vi "Parse URI.vi"(8 "error in (no error)":errorcluster, 11 "URI":string) -> (0 "error out":errorcluster, 3 "parsed URI":T1)   [LabVIEW 2020, in "NI_WFCN.lvlib"]
doc: "Parse a URI into its constituent parts. Component prefixes and suffixes denote presence:\n<b>suffixed user</b> ends with \"@\" if specified.\n<b>prefixed port</b> starts with \":\" if specified.\n<b>prefixed query</b> starts with \"?\" if specified.\n<b>prefixed fragment</b> starts with \"#\" if specified.\nIf a bare hostname is passed in, it will be returned in <b>undecoded.path</b>."
uses:
  <vilib>/net/WFCN/NI_WFCN.lvlib
  <vilib>/net/WFCN/Utility/URIv1.ctl
  <vilib>/net/WFCN/Utility/URI Path Components v1.ctl
  <vilib>/net/WFCN/Utility/URI Undecoded Components v1.ctl
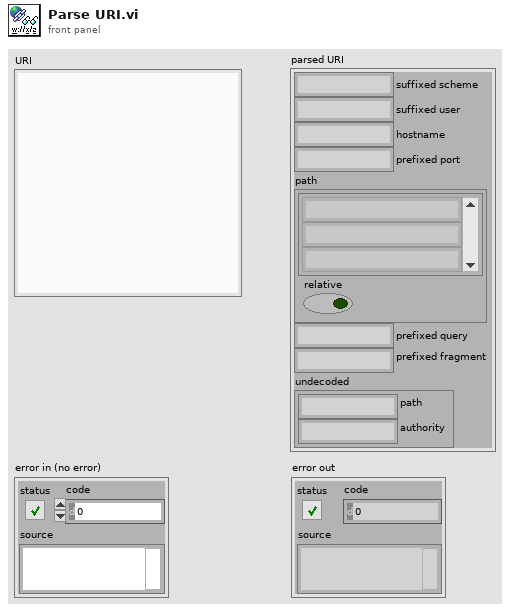
[diagram p1: front panel]
types:
  T1 = typedef "NI_WFCN.lvlib/URIv1.ctl" = cluster{"suffixed scheme":string, "suffixed user":string, "hostname":string, "prefixed port":string, "path":T2, "prefixed query":string, "prefixed fragment":string, "undecoded":T3}
  T2 = typedef "NI_WFCN.lvlib/URI Path Components v1.ctl" = cluster{"elements":string[], "relative":bool}
  T3 = typedef "NI_WFCN.lvlib/URI Undecoded Components v1.ctl" = cluster{"path":string, "authority":string}
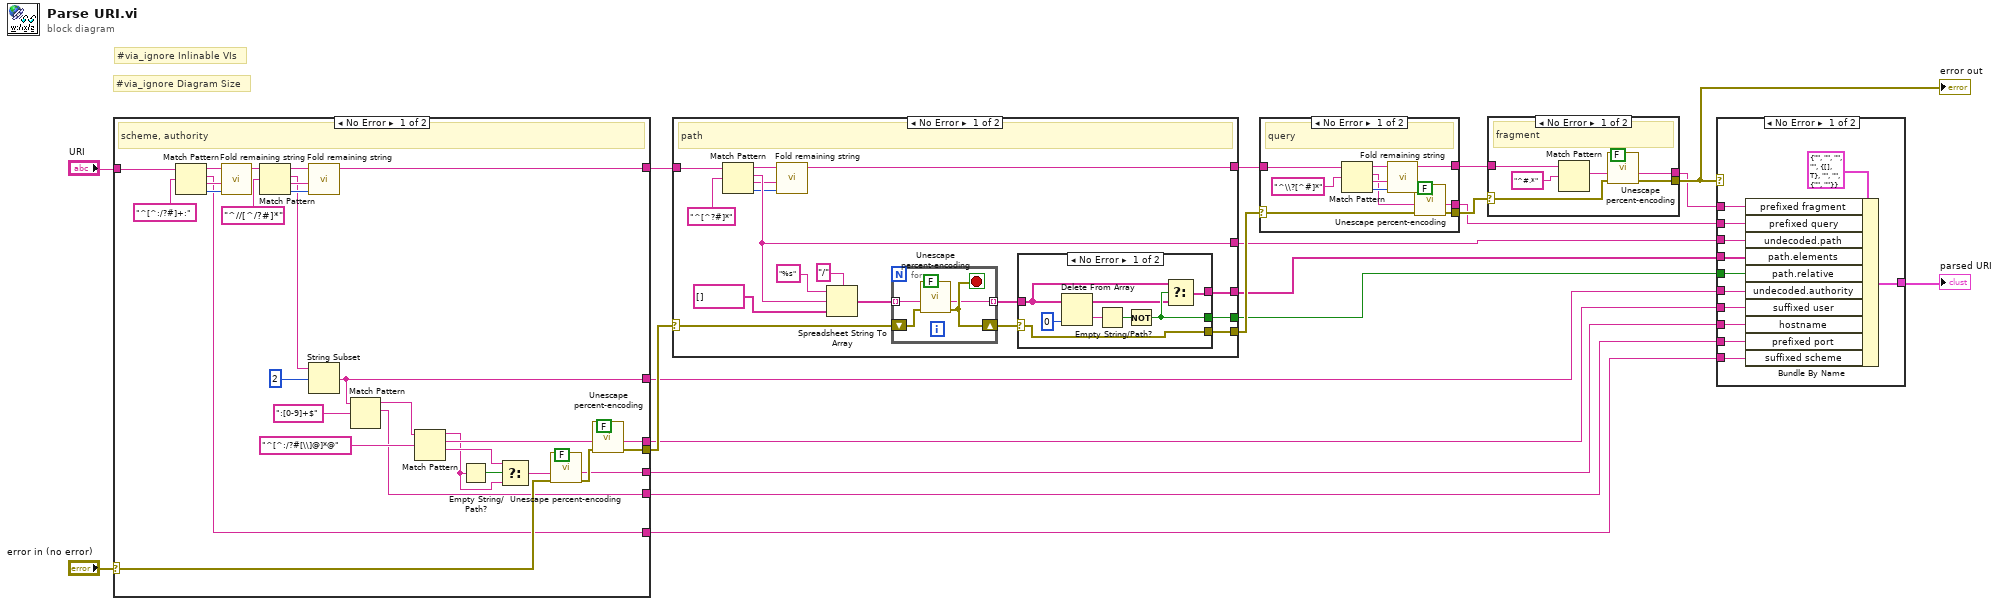
[diagram p0: block diagram]
diagram:
  # "#via_ignore Inlinable VIs"
  # "#via_ignore Diagram Size"
  n1 = case shown="No Error" "error in (no error)" {
    selector: "error in (no error)" -> [w32 w52]
    tunnel: "URI" -> [w51 _]
    tunnel: [w31 _] -> w15
    tunnel: [w30 w52] -> w16
    tunnel: [w29 _] -> w4
    tunnel: [w28 _] -> w3
    tunnel: [w27 _] -> w1
    tunnel: [w26 _] -> w2
    tunnel: [w25 _] -> w5
    frame No Error {
      # "scheme, authority"
      n2 = Match Pattern(string=w51, regular expression="^[^:/?#]+:") -> (before substring=w46:string, match substring=w27:string, after substring=w45:string, offset past match=w44:i32)  [unwired: 1 in]
      n3 = call <vilib>:"Fold remaining string.vi"("index"=w44, "after match"=w45, "before match"=w46) -> ("remaining"=w43:string)  [unwired: 4 in]
      n4 = Match Pattern(string=w43, regular expression="^//[^/?#]*") -> (before substring=w41:string, match substring=w37:string, after substring=w40:string, offset past match=w39:i32)  [unwired: 1 in]
      n5 = call <vilib>:"Fold remaining string.vi"("index"=w39, "after match"=w40, "before match"=w41) -> ("remaining"=w31:string)  [unwired: 4 in]
      n6 = String Subset(string=w37, offset (0)=2) -> (substring=w25:string)  [unwired: 1 in]
      n7 = Match Pattern(string=w25, regular expression=":[0-9]+$") -> (before substring=w48:string, match substring=w26:string)  [unwired: 1 in, 2 out]
      n8 = Match Pattern(string=w48, regular expression="^[^:/?#[\\]@]*@") -> (before substring=w22:string, match substring=w36:string, after substring=w23:string)  [unwired: 1 in, 1 out]
      n9 = Empty String/Path?(string/path=w22) -> (empty?=w24:bool)
      n10 = Select(t=w23, s=w24, f=w22) -> (s? t:f=w21:string)
      n11 = call <vilib>:"Unescape percent-encoding.vi"("percent-encoded string"=w21, "error in (no error)"=w32, "safe?"=FALSE) -> ("decoded string"=w28:string, "error out"=w35:errorcluster)  [unwired: 6 in]
      n12 = call <vilib>:"Unescape percent-encoding.vi"("percent-encoded string"=w36, "error in (no error)"=w35, "safe?"=FALSE) -> ("decoded string"=w29:string, "error out"=w30:errorcluster)  [unwired: 6 in]
    }
    frame Error {
    }
  }
  n13 = case shown="No Error" w16 {
    selector: w16 -> [w61 w84]
    tunnel: w15 -> [w62 _]
    tunnel: [w53 w84] -> w13
    tunnel: [w60 _] -> w6
    tunnel: [w59 _] -> w7
    tunnel: [w58 _] -> w8
    tunnel: [w54 _] -> w14
    frame No Error {
      # "path"
      n14 = Match Pattern(string=w62, regular expression="^[^?#]*") -> (before substring=w57:string, match substring=w58:string, after substring=w56:string, offset past match=w55:i32)  [unwired: 1 in]
      n15 = call <vilib>:"Fold remaining string.vi"("index"=w55, "after match"=w56, "before match"=w57) -> ("remaining"=w54:string)  [unwired: 4 in]
      n16 = Spreadsheet String To Array(delimiter (Tab)="/", format string="%s", spreadsheet string=w58, array type (2D Dbl)=string[] []) -> (array=w67:string[])
      n17 = for {
        tunnel: w67 -> [w81] mode=indexing
        shift-right: [w82] -> w68
        shift-left: w61 -> [w83]
        tunnel: [w80] -> w69 mode=indexing
        stop <- w82 stop-if-true
        n18 = call <vilib>:"Unescape percent-encoding.vi"("percent-encoded string"=w81, "error in (no error)"=w83, "safe?"=FALSE) -> ("decoded string"=w80:string, "error out"=w82:errorcluster)  [unwired: 6 in]
      }
      n19 = case shown="No Error" w68 {
        selector: w68 -> [w70 w78]
        tunnel: w69 -> [w72 _]
        tunnel: [w70 w78] -> w53
        tunnel: [w74 _] -> w59
        tunnel: [w73 _] -> w60
        frame No Error {
          n20 = Delete From Array(array=w72, index=0) -> (deleted portion=w76:string, array with subset deleted=w71:string[])  [unwired: 1 in]
          n21 = Empty String/Path?(string/path=w76) -> (empty?=w75:bool)
          n22 = Not(x=w75) -> (.not. x?=w73:bool)
          n23 = Select(t=w72, s=w73, f=w71) -> (s? t:f=w74:string[])
        }
        frame Error {
        }
      }
    }
    frame Error {
    }
  }
  n24 = case shown="No Error" w13 {
    selector: w13 -> [w88 w96]
    tunnel: w14 -> [w89 _]
    tunnel: [w87 _] -> w11
    tunnel: [w86 w96] -> w12
    tunnel: [w85 _] -> w9
    frame No Error {
      # "query"
      n25 = Match Pattern(string=w89, regular expression="^\\?[^#]*") -> (before substring=w94:string, match substring=w91:string, after substring=w93:string, offset past match=w92:i32)  [unwired: 1 in]
      n26 = call <vilib>:"Fold remaining string.vi"("index"=w92, "after match"=w93, "before match"=w94) -> ("remaining"=w87:string)  [unwired: 4 in]
      n27 = call <vilib>:"Unescape percent-encoding.vi"("percent-encoded string"=w91, "error in (no error)"=w88, "safe?"=FALSE) -> ("decoded string"=w85:string, "error out"=w86:errorcluster)  [unwired: 6 in]
    }
    frame Error {
    }
  }
  n28 = case shown="No Error" w12 {
    selector: w12 -> [w100 w104]
    tunnel: w11 -> [w99 _]
    tunnel: [w98 _] -> w10
    tunnel: [w97 w104] -> w17
    frame No Error {
      # "fragment"
      n29 = Match Pattern(string=w99, regular expression="^#.*") -> (match substring=w102:string)  [unwired: 1 in, 3 out]
      n30 = call <vilib>:"Unescape percent-encoding.vi"("percent-encoded string"=w102, "error in (no error)"=w100, "safe?"=FALSE) -> ("decoded string"=w98:string, "error out"=w97:errorcluster)  [unwired: 6 in]
    }
    frame Error {
    }
  }
  "error out" <- w17
  n31 = case shown="No Error" w17 {
    tunnel: w10 -> [w115 _]
    tunnel: w9 -> [w114 _]
    tunnel: w8 -> [w113 _]
    tunnel: w7 -> [w112 _]
    tunnel: w6 -> [w111 _]
    tunnel: [w110 _] -> w18
    tunnel: w5 -> [w109 _]
    tunnel: w4 -> [w108 _]
    tunnel: w3 -> [w107 _]
    tunnel: w2 -> [w106 _]
    tunnel: w1 -> [w105 _]
    frame No Error {
      n32 = Bundle By Name(cluster=T1 {"suffixed scheme"="", "suffixed user"="", "hostname"="", "prefixed port"="", "path"={"elements"=[], "relative"=TRUE}, "prefixed query"="", "prefixed fragment"="", "undecoded"={"path"="", "authority"=""}}, "prefixed fragment"=w115, "prefixed query"=w114, "undecoded.path"=w113, "path.elements"=w112, "path.relative"=w111, "undecoded.authority"=w109, "suffixed user"=w108, "hostname"=w107, "prefixed port"=w106, "suffixed scheme"=w105) -> (w110:T1)
    }
    frame Error {
    }
  }
  "parsed URI" <- w18
